vi "testing sector pixel.vi"() -> ()   [LabVIEW 2013]
uses:
  FPGA Image Processing.lvlib
  <vilib>/Platform/TimedLoop/XDataNode/XDataNode.xnode
  <vilib>/Platform/TimedLoop/XDataNode/nitl_modes.ctl
  <vilib>/Platform/TimedLoop/XDataNode/XDNodeRunTimeDep.lvlib
  <vilib>/Platform/TimedLoop/XDataNode/wakeup.ctl
  <vilib>/Platform/TimedLoop/XDataNode/timing_clust.ctl
  Sector/Accumulate/Sector Parameter Cluster.ctl
panel:
  out "output valid":bool
  out "Numeric":i32
  in  "stop":bool
  out "sector #":u8
  in  "Sector Parameters":T1={"Start Angle"=0.08990478515625, "End Angle"=0.2884521484375, "Inner Radius"=309, "Outter Radius"=405, "Hinge X"=1057, "Hinge Y"=785, "NumWingSectors"=8}
  in  "Pixel Y":u16=553
  in  "Pixel X":u16=1295
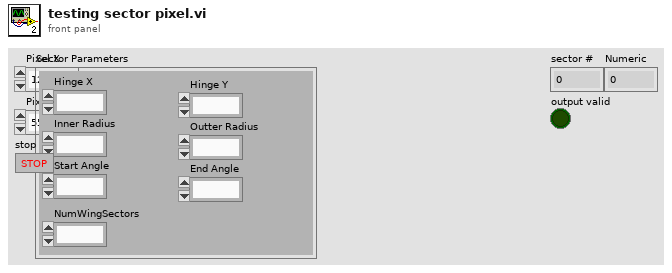
[diagram p1: front panel]
types:
  T1 = typedef "Sector Parameter Cluster.ctl" = cluster{"Start Angle":fxp<+/-,17,2>, "End Angle":fxp<+,17,3>, "Inner Radius":u16, "Outter Radius":u16, "Hinge X":u16, "Hinge Y":u16, "NumWingSectors":u8}
  T2 = typedef "XDNodeRunTimeDep.lvlib/timing_clust.ctl" = cluster{"Expected End [f-1]":u64, "Actual End [f-1]":u64, "Finished Late? [f-1]":bool, "Expected End [i-1]":u64, "Actual End [i-1]":u64, "Finished Late? [i-1]":bool, "Expected Start [i]":u64, "Actual Start [i]":u64, "Expected Start [f]":u64, "Actual Start [f]":u64, "Source Name":string, "Structure Name":string, "Period":i64, "Deadline":i64, "Offset":i64, "Start":i64, "Priority":i32, "Timeout":i32, "Mode":T3, "Wakeup Reason":T4, "Error":errorcluster, "Source Type":string, "Secondary Source Type":string, "Global End Time":u64, "Global Start Time":u64, "Frame Duration":u64, "Iteration Duration":u64, "Assigned CPU":i32, "I/O Scan Engine Mode":u32}
  T3 = typedef "XDNodeRunTimeDep.lvlib/nitl_modes.ctl" = enum32{"No Change", "Process missed periods, maintain original phase", "Discard missed periods, maintain original phase", "Process missed periods, ignore original phase", "Discard missed periods, ignore original phase"}
  T4 = typedef "XDNodeRunTimeDep.lvlib/wakeup.ctl" = enum32{"Normal", "Aborted", "Asynchronous wakeup", "Timing source error", "Timed loop error", "Timeout"}
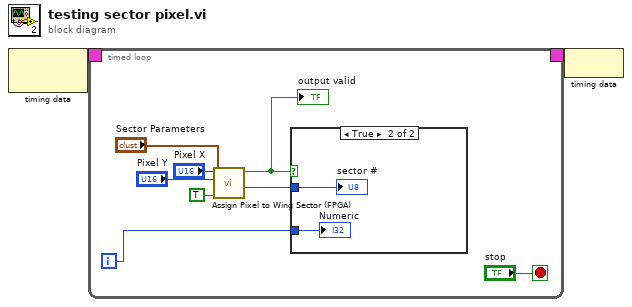
[diagram p0: block diagram]
diagram:
  n1 = node-c288() -> (w2:T2)  [unwired: 1 in]
  n2 = timed-loop {
    timing: w2 -> [_]
    timing-out: [_] -> w1
    i -> [w3]
    stop <- "stop" stop-if-true
    n3 = call "Assign Pixel to Wing Sector (FPGA).vi"("Right Wing?"=TRUE, "Sector Parameters"="Sector Parameters", "Pixel Y"="Pixel Y", "Pixel X"="Pixel X") -> ("Pixel Intensity Out"=w6:u8, "output valid"=w5:bool)  [unwired: 4 in, 1 out]
    "output valid" <- w5
    n4 = case shown="True" w5 {
      tunnel: w6 -> [_ w12]
      tunnel: w3 -> [_ w11]
      frame False {
      }
      frame True {
        "sector #" <- w12
        "Numeric" <- w11
      }
    }
  }
  n5 = node-c288(w1) -> ()
